vi "Read Value.vi"(8 "error in (no error)":errorcluster, 11 "int32 in":refnum<class "bool.lvclass">) -> (0 "error out":errorcluster, 2 "Value":bool, 3 "int32 out":refnum<class "bool.lvclass">)   [LabVIEW 2020, in "Protobuf RAW.lvlib" / "bool.lvclass"]
uses:
  bool.lvclass
  bool.lvclass/bool.ctl
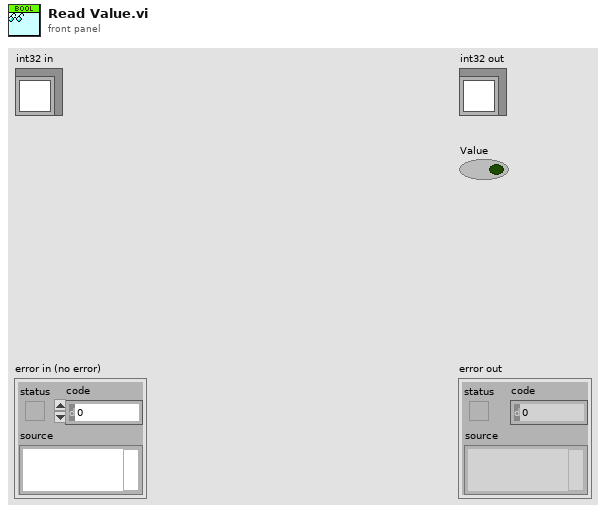
[diagram p1: front panel]
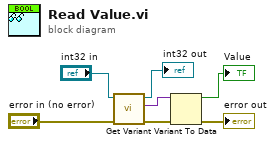
[diagram p0: block diagram]
diagram:
  n1 = call-dynamic "Get Variant.vi"("error in (no error)"="error in (no error)", "int32 in"="int32 in") -> ("error out"=w6:errorcluster, "Variant"=w2:variant, "int32 out"=→"int32 out":refnum<class "bool.lvclass">)  [unwired: 7 in]
  n2 = Variant To Data(error in=w6, Variant=w2) -> (data=→"Value":bool, error out=→"error out":errorcluster)  [unwired: 1 in]
